vi "Handle Actor Core Events.vi"(8 "error in (no error)":errorcluster, 11 "ActorAutoRegistration":refnum<class "ActorAutoRegistration.lvclass">) -> (0 "error out":errorcluster)   [LabVIEW 2015, in "ActorEvents.lvlib" / "ActorAutoRegistration.lvclass"]
doc: "<License>\nCopyright © 2017 Composed Systems, LLC | All rights reserved\nwww.composed.io\n\nAuthor: Ethan Stern <ethan.stern@composed.io>\n\nThis software is provided \"AS IS\" WITHOUT WARRANTIES, either express or implied, AND IS FOR EDUCATIONAL PURPOSES ONLY.\n</License>"
uses:
  ActorAutoRegistration.lvclass
  ActorAutoRegistration.lvclass/ActorAutoRegistration.ctl
  ActorAutoRegistration Messages/PanelCloseMsg/PanelCloseMsg.lvclass
  ActorAutoRegistration Messages/ValueChangeMsg/ValueChangeMsg.lvclass
  ActorAutoRegistration Messages/ControlMouseUpMsg/ControlMouseUpMsg.lvclass
  ActorAutoRegistration Messages/ControlMouseDownMsg/ControlMouseDownMsg.lvclass
  ActorAutoRegistration Messages/UserMenuSelectionMsg/UserMenuSelectionMsg.lvclass
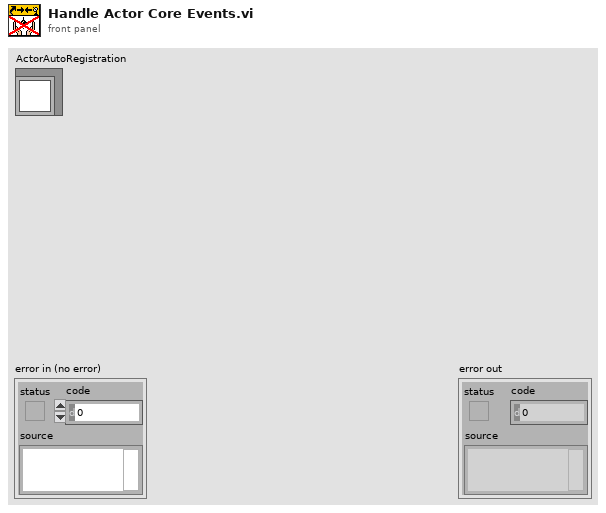
[diagram p1: front panel]
types:
  T1 = typedef "AutoRegistration.lvlib/AutoRegistration.lvclass/Auto-Event Registration Refnum.ctl" = refnum<event-registration>
  T2 = typedef "LVPoint32TypeDef.ctl" = cluster{"Horizontal":i32, "Vertical":i32}
  T3 = cluster{"Shift":bool, "Ctrl":bool, "Alt":bool, "Cmd":bool, "Opt":bool}
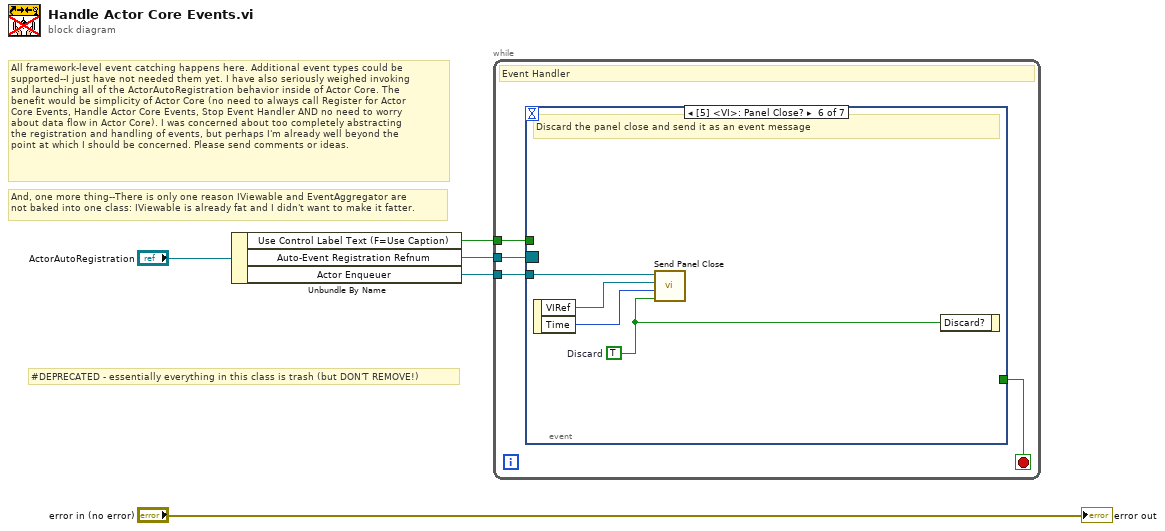
[diagram p0: block diagram]
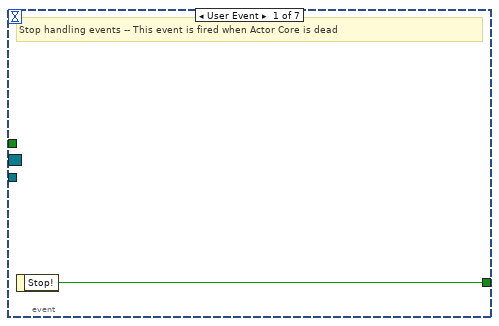
[diagram p2: hidden frame]
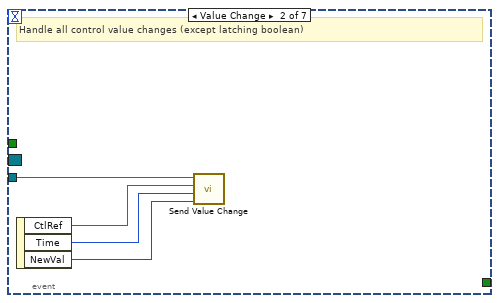
[diagram p3: hidden frame]
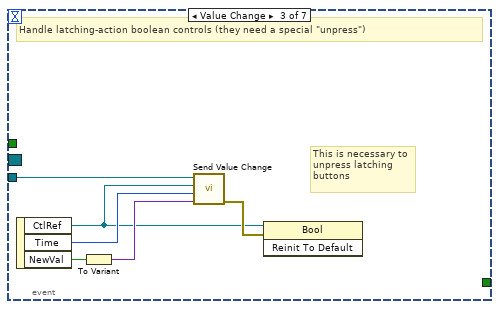
[diagram p4: hidden frame]
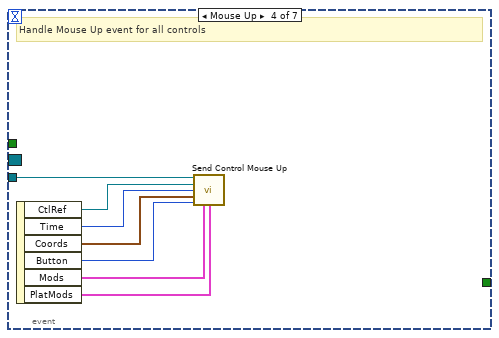
[diagram p5: hidden frame]
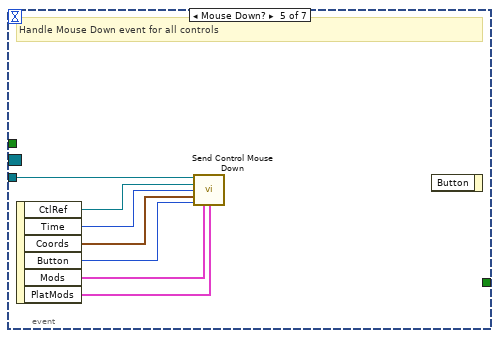
[diagram p6: hidden frame]
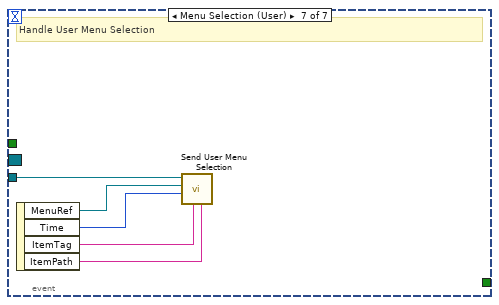
[diagram p7: hidden frame]
diagram:
  # "#DEPRECATED - essentially everything in this class is trash (but DON'T REMOVE!)"
  # "And, one more thing--There is only one reason IViewable and EventAggregator are\nnot baked into one class: IViewable is already fat and I didn't want to make it fatter."
  # "All framework-level event catching happens here. Additional event types could be\nsupported--I just have not needed them yet. I have also seriously weighed invoking\nand launching all of the ActorAutoRegistration behavior inside of Actor Core. The\nbenefit would be simplicity of Actor Core (no need to always call Register for Actor\nCore Events, Handle Actor Core Events, Stop Event Handler AND no need to worry\nabout data flow in Actor Core). I was concerned about too completely abstracting\nthe registration and handling of events, but perhaps I'm already well beyond the\npoint at which I should be concerned. Please send comments or ideas."
  n1 = Unbundle By Name("ActorAutoRegistration") -> ("Use Control Label Text (F=Use Caption)"=w2:bool, "Auto-Event Registration Refnum"=w1:T1, "Actor Enqueuer"=w3:refnum<class "Message Enqueuer.lvclass">)
  n2 = while {
    tunnel: w3 -> [w8]
    tunnel: w2 -> [w7]
    tunnel: w1 -> [w6]
    stop <- w9 stop-if-true
    # "Event Handler"
    n3 = event shown="[5] <VI>: Panel Close?" {
      selector: w6 -> [_ _ _ _ _ _ _]
      dyn-events: _ -> [_ _ _ _ _ _ _]
      timeout: _ -> [_ _ _ _ _ _ _]
      tunnel: [w10 _ _ _ _ _ _] -> w9
      tunnel: w8 -> [_ w14 w20 w27 w34 w38 w43]
      tunnel: w7 -> [_ _ _ _ _ _ _]
      event User Event {
        # "Stop handling events -- This event is fired when Actor Core is dead"
        n4 = event-data() -> ("Stop!"=w10:bool)  [unwired: 1 in]
      }
      event Value Change {
        # "Handle all control value changes (except latching boolean)"
        n5 = event-data() -> ("CtlRef"=w13:refnum<vi>, "Time"=w12:u32, "NewVal"=w11:variant)  [unwired: 1 in]
        n6 = call "Send Value Change.vi"("New Value"=w11, "Time"=w12, "Ctl Refnum"=w13, "Message Enqueuer in"=w14) -> ()  [unwired: 7 in, 1 out]
      }
      event Value Change {
        # "This is necessary to\nunpress latching\nbuttons"
        # "Handle latching-action boolean controls (they need a special \"unpress\")"
        n7 = event-data() -> ("CtlRef"=w15:refnum<vi>, "Time"=w17:u32, "NewVal"=w19:bool)  [unwired: 1 in]
        n8 = To Variant(anything=w19) -> (Variant=w16:variant)
        n9 = call "Send Value Change.vi"("New Value"=w16, "Time"=w17, "Ctl Refnum"=w15, "Message Enqueuer in"=w20) -> ("error out"=w18:errorcluster)  [unwired: 7 in]
        n10 = invoke class="Bool" method="Reinit To Default"(reference=w15, error in=w18) -> ()  [unwired: 1 in, 3 out]
      }
      event Mouse Up {
        # "Handle Mouse Up event for all controls"
        n11 = event-data() -> ("CtlRef"=w26:refnum<vi>, "Time"=w25:u32, "Coords"=w24:T2, "Button"=w23:u16, "Mods"=w22:cluster{"Double Click":bool, "Menu Key":bool}, "PlatMods"=w21:T3)  [unwired: 1 in]
        n12 = call "Send Control Mouse Up.vi"("Message Enqueuer in"=w27, "Ctl Refnum"=w26, "Time"=w25, "Coords"=w24, "Button"=w23, "Mods"=w22, "PlatMods"=w21) -> ()  [unwired: 8 in, 1 out]
      }
      event Mouse Down? {
        # "Handle Mouse Down event for all controls"
        n13 = event-data() -> ("CtlRef"=w33:refnum<vi>, "Time"=w32:u32, "Coords"=w31:T2, "Button"=w30:u16, "Mods"=w29:cluster{"Double Click":bool, "Menu Key":bool}, "PlatMods"=w28:T3)  [unwired: 1 in]
        n14 = call "Send Control Mouse Down.vi"("Message Enqueuer in"=w34, "Ctl Refnum"=w33, "Time"=w32, "Coords"=w31, "Button"=w30, "Mods"=w29, "PlatMods"=w28) -> ()  [unwired: 8 in, 1 out]
        n15 = event-data() -> ()  [unwired: 2 in, 1 out]
      }
      event Panel Close? {
        w36 = TRUE  # Discard
        # "Discard the panel close and send it as an event message"
        n16 = event-data() -> ("VIRef"=w37:refnum<vi>, "Time"=w35:u32)  [unwired: 1 in]
        n17 = call "Send Panel Close.vi"("Discarded?"=w36, "Time"=w35, "VI Refnum"=w37, "Message Enqueuer in"=w38) -> ()  [unwired: 7 in, 1 out]
        n18 = event-data("Discard?"=w36) -> ()  [unwired: 1 in, 1 out]
      }
      event Menu Selection (User) {
        # "Handle User Menu Selection"
        n19 = event-data() -> ("MenuRef"=w42:refnum<k9>, "Time"=w41:u32, "ItemTag"=w40:string, "ItemPath"=w39:string)  [unwired: 1 in]
        n20 = call "Send User Menu Selection.vi"("Item Path"=w39, "Item Tag"=w40, "Time"=w41, "MenuRef"=w42, "Message Enqueuer in"=w43) -> ()  [unwired: 6 in, 1 out]
      }
    }
  }
  "error out" <- "error in (no error)"
